vi "fisiere_v6.vi"() -> ()   [LabVIEW 2009]
panel:
  out "txt_wr":string
  out "calc":bool
  in  "Flag":u8
  in  "Nr_win":u8=4 max=10 step=1
  out "Participants":string[][](array[string])
  in  "Path to results file":path=path "E:/Projects/Lab_view/Proiecte_concurs/Project 4/Winners.txt"
  out "Winners":string[][](array[string])
  out "win_i":u8[](array[numeric])=[1, 4, 0, 2]
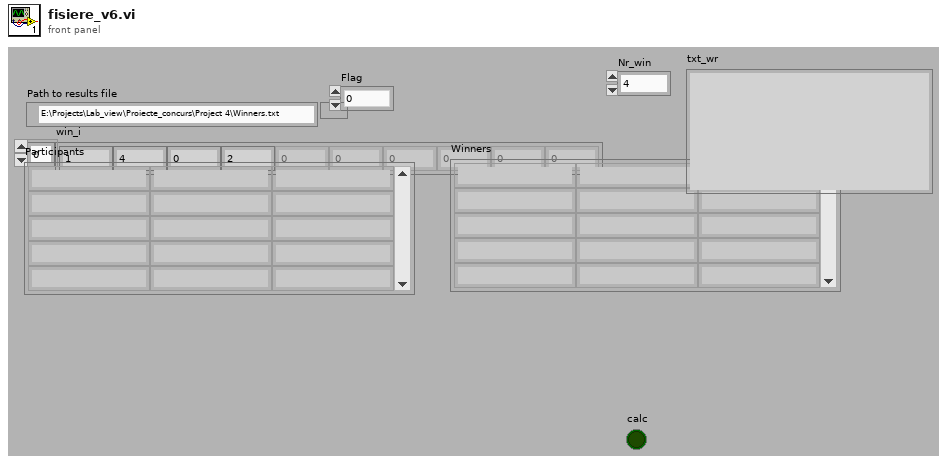
[diagram p1: front panel]
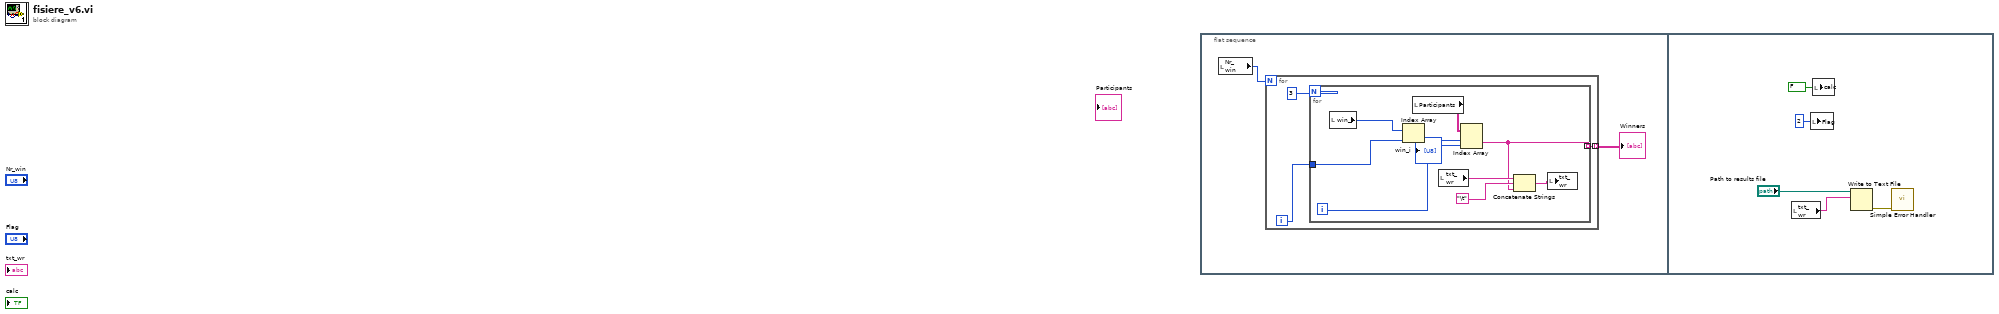
[diagram p0: block diagram]
diagram:
  n1 = flat-sequence {
    frame #0 {
      n2 = local read "Nr_win"() -> (w1:u8)
      n3 = for {
        N: w1 -> [_]
        tunnel: [w5] -> w2 mode=indexing
        i -> [w4]
        n4 = for {
          N: 3 -> [_]
          tunnel: [w6] -> w5 mode=indexing
          tunnel: w4 -> [w12]
          i -> [w10]
          n5 = local read "win_i"() -> (w13:u8[])
          n6 = Index Array(array=w13, index=w12) -> (element=w11:u8)
          n7 = local read "Participants"() -> (w14:string[][])
          n8 = local read "txt_wr"() -> (w8:string)
          n9 = Index Array(array=w14, index (row)=w11, index (col)=w10) -> (element=w6:string)
          n10 = Concatenate Strings(w8, "\t", w6) -> (w9:string)
          n11 = local write "txt_wr"(w9) -> ()
        }
      }
      "Winners" <- w2
    }
    frame #1 {
      n12 = local read "txt_wr"() -> (w15:string)
      n13 = local write "Flag"(u8 2 ("Flag")) -> ()
      n14 = local write "calc"(FALSE ("calc")) -> ()
      n15 = Write to Text File(file (use dialog)="Path to results file", text=w15) -> (error out=w16:errorcluster)  [unwired: 2 in, 2 out]
      n16 = call <vilib>:"Simple Error Handler.vi"("error in (no error)"=w16) -> ()  [unwired: 4 in, 5 out]
    }
  }
